vi "sequence sort unknown.vi"() -> ()   [LabVIEW 2016]
uses:
  controls/data control cluster.ctl
panel:
  in  "DATA CLUSTER in":T1
  out "output cluster":T1
  out "Array 3":dbl[][](array[numeric])
  out "cycle result header":string[](array[string])
  out "Array 2":i32[](array[numeric])
  out "Cycle data":dbl[][][](array[numeric])
  out "Numeric 2":i32
  out "Numeric":i32
  out "Array":dbl[][](array[numeric])
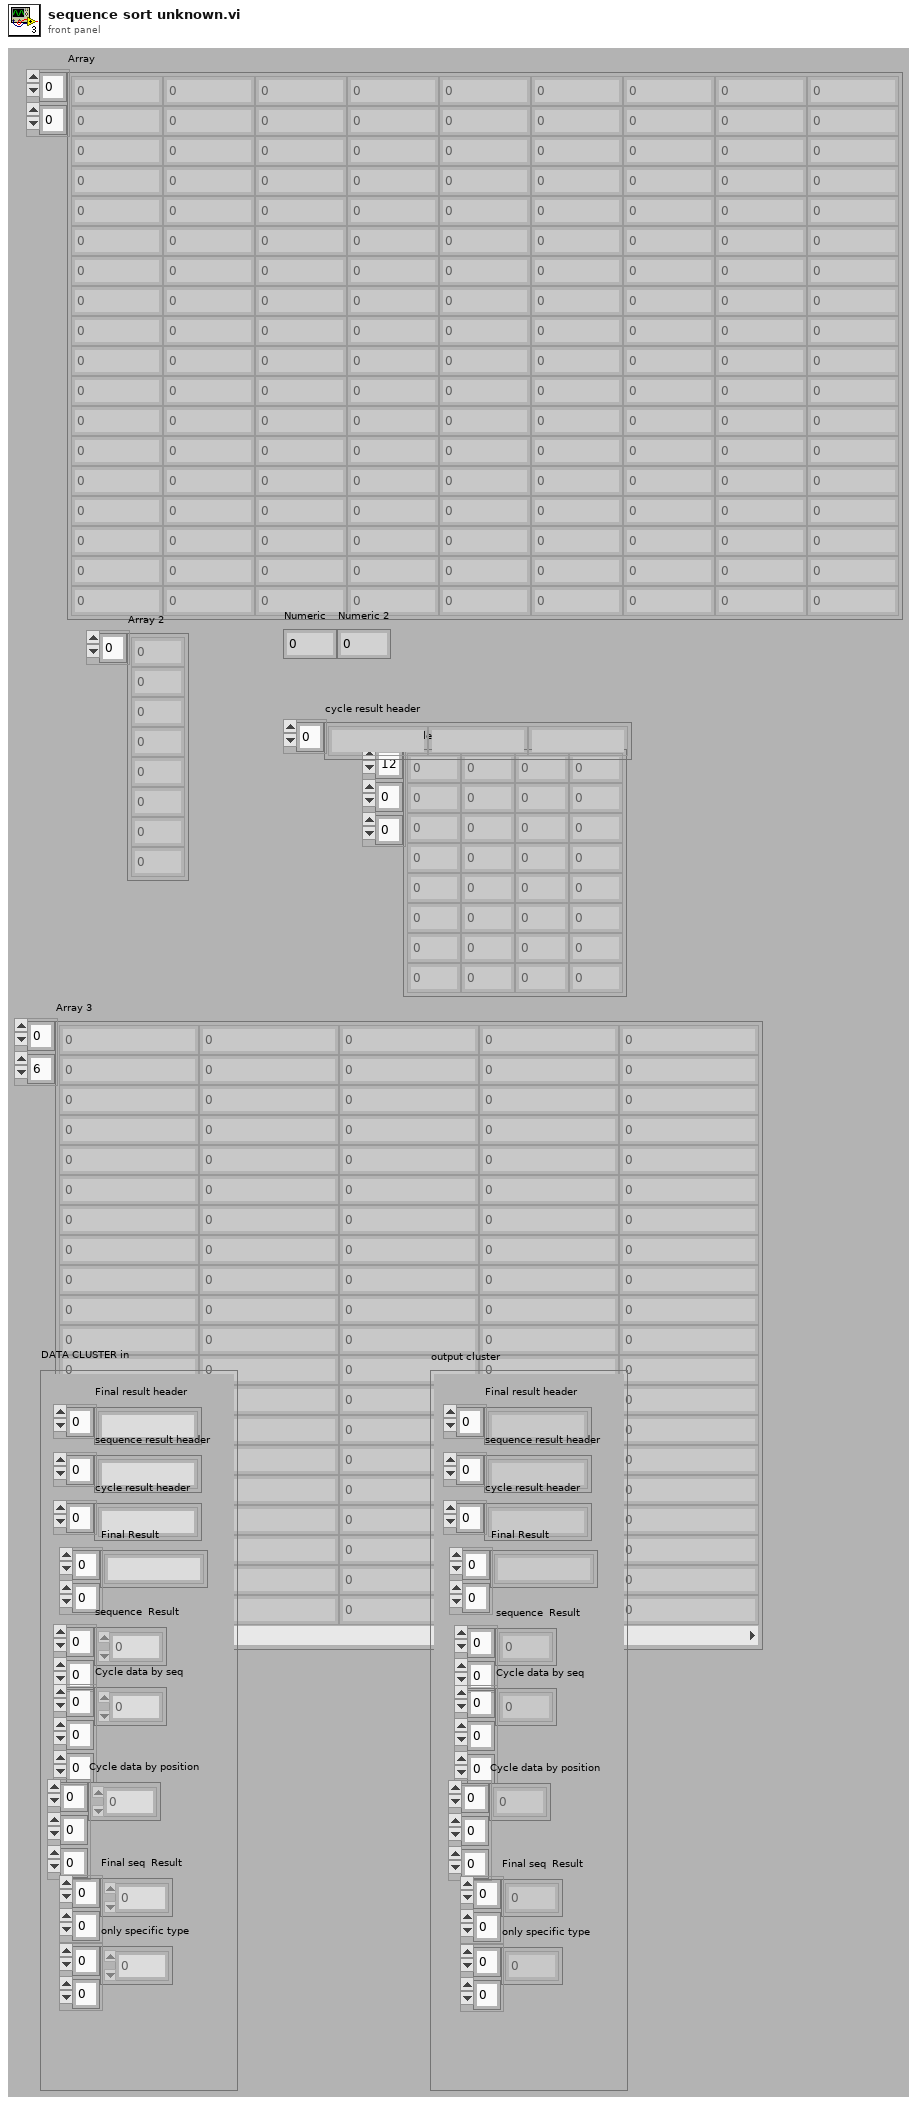
[diagram p1: front panel]
types:
  T1 = typedef "data control cluster.ctl" = cluster{"Final result header":string[], "sequence result header":string[], "cycle result header ":string[], "Final Result":string[][], "sequence  Result":dbl[][], "Cycle data by seq":dbl[][][], "Cycle data by position":dbl[][][], "Final seq  Result":dbl[][], "only specific type":dbl[][]}
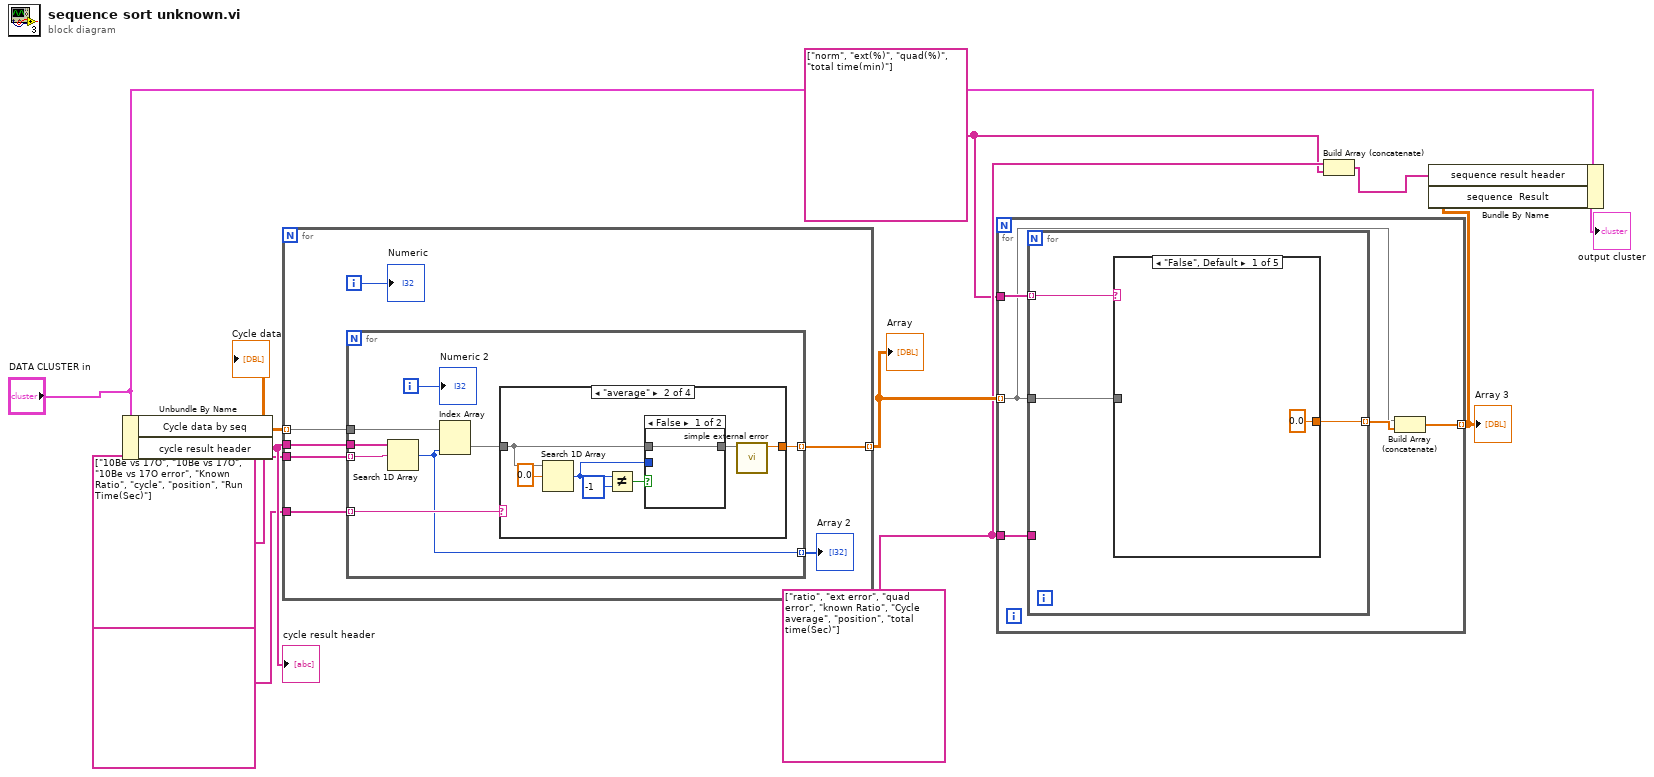
[diagram p0: block diagram]
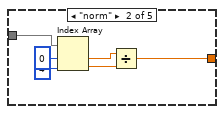
[diagram p2: hidden frame]
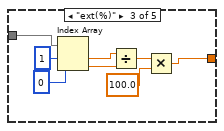
[diagram p3: hidden frame]
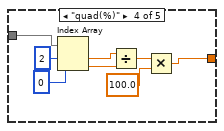
[diagram p4: hidden frame]
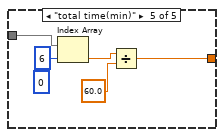
[diagram p5: hidden frame]
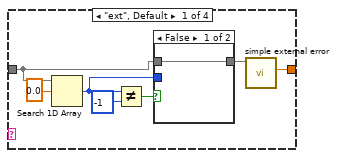
[diagram p6: hidden frame]
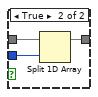
[diagram p7: hidden frame]
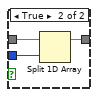
[diagram p8: hidden frame]
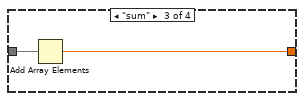
[diagram p9: hidden frame]
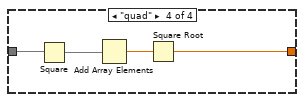
[diagram p10: hidden frame]
diagram:
  w6 = string[] ["ratio", "ext error", "quad error", "known Ratio", "Cycle average", "position", "total time(Sec)"]
  w5 = string[] ["norm", "ext(%)", "quad(%)", "total time(min)"]
  n1 = Unbundle By Name("DATA CLUSTER in") -> ("Cycle data by seq"=w11:dbl[][][], "cycle result header"=w10:string[])
  "Cycle data" <- w11
  "cycle result header" <- w10
  n2 = for {
    tunnel: w11 -> [w16] mode=indexing
    tunnel: w10 -> [w18]
    tunnel: string[] ["10Be vs 17O", "10Be vs 17O", "10Be vs 17O error", "Known Ratio", "cycle", "position", "Run Time(Sec)"] -> [w17]
    tunnel: string[] ["average", "ext", "quad", "average", "average", "average", "sum"] -> [w15]
    tunnel: [w14] -> w7 mode=indexing
    i -> [w13]
    n3 = for {
      tunnel: w18 -> [w26]
      tunnel: w17 -> [w25] mode=indexing
      tunnel: w16 -> [w24]
      tunnel: w15 -> [w23] mode=indexing
      tunnel: [w21] -> w14 mode=indexing
      tunnel: [w19] -> w12 mode=indexing
      i -> [w20]
      n4 = Search 1D Array(1D array=w26, element=w25) -> (index of element=w19:i32)  [unwired: 1 in]
      n5 = Index Array(array=w24, index (col)=w19) -> (element=w22:dbl[])  [unwired: 1 in]
      n6 = case shown="\"average\"" w23 {
        tunnel: w22 -> [w31 w42 w50 w54]
        tunnel: [w33 w44 w49 w51] -> w21
        frame "ext", Default {
          n7 = Search 1D Array(1D array=w31, element=0.0) -> (index of element=w28:i32)  [unwired: 1 in]
          n8 = Not Equal?(x=w28, y=-1) -> (x != y?=w29:bool)
          n9 = case shown="False" w29 {
            tunnel: w28 -> [_ w37]
            tunnel: w31 -> [w34 w36]
            tunnel: [w34 w35] -> w30
            frame False {
            }
            frame True {
              n10 = Split 1D Array(array=w36, index=w37) -> (first subarray=w35:dbl[])  [unwired: 1 out]
            }
          }
          n11 = call "simple external error.vi"("cycle results"=w30) -> ("External error"=w33:dbl)  [unwired: 7 in, 3 out]
        }
        frame "average" {
          n12 = Search 1D Array(1D array=w42, element=0.0) -> (index of element=w39:i32)  [unwired: 1 in]
          n13 = Not Equal?(x=w39, y=-1) -> (x != y?=w40:bool)
          n14 = case shown="False" w40 {
            tunnel: w39 -> [_ w48]
            tunnel: w42 -> [w45 w47]
            tunnel: [w45 w46] -> w41
            frame False {
            }
            frame True {
              n15 = Split 1D Array(array=w47, index=w48) -> (first subarray=w46:dbl[])  [unwired: 1 out]
            }
          }
          n16 = call "simple external error.vi"("cycle results"=w41) -> ("Sequence result"=w44:dbl)  [unwired: 7 in, 3 out]
        }
        frame "sum" {
          n17 = Add Array Elements(numeric array=w50) -> (sum=w49:dbl)
        }
        frame "quad" {
          n18 = Square(x=w54) -> (x^2=w53:dbl[])
          n19 = Add Array Elements(numeric array=w53) -> (sum=w52:dbl)
          n20 = Square Root(x=w52) -> (sqrt(x)=w51:dbl)
        }
      }
      "Numeric 2" <- w20
    }
    "Array 2" <- w12
    "Numeric" <- w13
  }
  "Array" <- w7
  n21 = for {
    tunnel: w7 -> [w56] mode=indexing
    tunnel: w5 -> [w59]
    tunnel: w6 -> [w58]
    tunnel: [w55] -> w2 mode=indexing
    n22 = for {
      tunnel: w59 -> [w62] mode=indexing
      tunnel: w58 -> [_]
      tunnel: w56 -> [w61]
      tunnel: [w60] -> w57 mode=indexing
      n23 = case shown="\"False\", Default" w62 {
        tunnel: w61 -> [_ w69 w77 w85 w90]
        tunnel: [0.0 w64 w70 w78 w86] -> w60
        frame "False", Default {
        }
        frame "norm" {
          n24 = Index Array(array=w69, index #1=0 ("index"), index #2=4 ("index")) -> (element #1=w65:dbl, element #2=w66:dbl)
          n25 = Divide(x=w65, y=w66) -> (x/y=w64:dbl)
        }
        frame "ext(%)" {
          n26 = Index Array(array=w77, index #1=1 ("index"), index #2=0 ("index")) -> (element #1=w73:dbl, element #2=w74:dbl)
          n27 = Divide(x=w73, y=w74) -> (x/y=w72:dbl)
          n28 = Multiply(x=w72, y=100.0) -> (x*y=w70:dbl)
        }
        frame "quad(%)" {
          n29 = Index Array(array=w85, index #1=2 ("index"), index #2=0 ("index")) -> (element #1=w81:dbl, element #2=w82:dbl)
          n30 = Divide(x=w81, y=w82) -> (x/y=w80:dbl)
          n31 = Multiply(x=w80, y=100.0) -> (x*y=w78:dbl)
        }
        frame "total time(min)" {
          (unwired) 0 ("index")
          n32 = Index Array(array=w90, index=6) -> (element=w88:dbl)
          n33 = Divide(x=w88, y=60.0) -> (x/y=w86:dbl)
        }
      }
    }
    n34 = Build Array (concatenate)(w56, w57) -> (w55:dbl[])
  }
  "Array 3" <- w2
  n35 = Build Array (concatenate)(w6, w5) -> (w3:string[])
  n36 = Bundle By Name(cluster="DATA CLUSTER in", "sequence result header"=w3, "sequence  Result"=w2) -> (→"output cluster":T1)
